vi "Tosca-Trace-Logging Thread.vi"(7 "IPC":T1) -> ()   [LabVIEW 2020]
uses:
  IPC VIs/Tosca-IPC.ctl
  Classes/Parameters/Parameters.lvclass
  Digital Input VIs/Tosca-DI Queue Data.ctl
  Digital Input VIs/Tosca-Input Event.ctl
  Digital Input VIs/Tosca-Input Criterion.ctl
  epl-vi-lib/Utility VIs/Type Defs/Logic State.ctl
  Typedefs/Tosca-Accumulator.ctl
  Typedefs/Tosca-State AODO.ctl
  Typedefs/Tosca-AO Runtime.ctl
  Typedefs/Tosca-DO Runtime.ctl
  epl-vi-lib/Signal Synthesis VIs/4th Generation/Classes/SignalManager/SignalManager.lvclass
  Typedefs/Tosca-Synapse Start Data.ctl
  IPC VIs/Tosca-Message.ctl
  IPC VIs/Tosca-Message Action.ctl
  Typedefs/Tosca-Thread Type.ctl
  Imaging VIs/Tosca-2P-Notifier Data.ctl
  Typedefs/Tosca-MATLAB Queue Data.ctl
  Visual Stim VIs/Tosca-Grating.ctl
  Visual Stim VIs/Tosca-Grating Type.ctl
  Typedefs/Tosca-File IO Notification.ctl
  Tosca-Trace Data.ctl
  Tosca-Trace-Event.ctl
  <vilib>/Utility/error.llb/Error Cluster From Error Code.vi
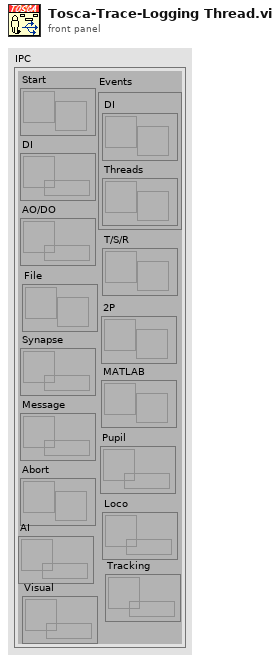
[diagram p1: front panel]
types:
  T1 = typedef "Tosca-IPC.ctl" = cluster{"Start":refnum<notifier>, "DI":refnum<queue>, "AO/DO":refnum<queue>, "Synapse":refnum<queue>, "Message":refnum<queue>, "Abort":refnum<notifier>, "Events":cluster{"DI":refnum<user-event>, "Threads ":refnum<user-event>}, "T/S/R":refnum<notifier>, "2P":refnum<notifier>, "MATLAB":refnum<notifier>, "Pupil":refnum<queue>, "Loco":refnum<queue>, "AI":refnum<queue>, "Tracking":refnum<queue>, "Visual":refnum<queue>, "File":refnum<notifier>}
  T2 = typedef "Tosca-Trace Data.ctl" = cluster{"Time":dbl, "Event":T3, "Source":string, "Message":string, "Data":dbl}
  T3 = typedef "Tosca-Trace-Event.ctl" = enum16{"Unspecified", "Trial start", "Enqueue", "Result", "End parser", "Frame", "Queue available", "Timeout sent", "WritePos", "TTL"}
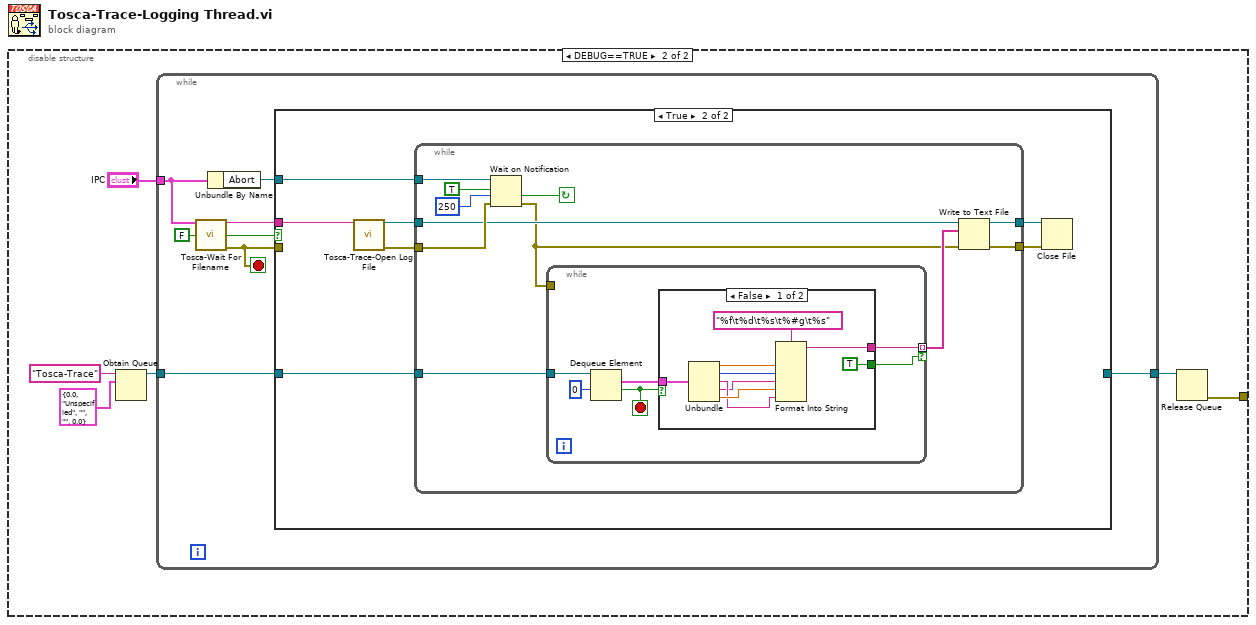
[diagram p0: block diagram]
diagram:
  n1 = disable-structure shown="DEBUG==TRUE" {
    disable-tunnel: [_ w1] -> _
    frame condition #0 {
    }
    frame condition #1 (active) {
      n2 = Obtain Queue(name (unnamed)="Tosca-Trace", element data type=T2 {"Time"=0.0, "Event"=enum."Unspecified", "Source"="", "Message"="", "Data"=0.0} ("Trace Data")) -> (queue out=w3:refnum<queue>)  [unwired: 3 in, 2 out]
      n3 = while {
        tunnel: w3 -> [w14]
        tunnel: [w13] -> w6
        tunnel: "IPC" -> [w10]
        stop <- w8 stop-if-true
        n4 = call "Tosca-Wait For Filename.vi"("IPC"=w10, "Times out?"=FALSE ("Time out?")) -> ("Filestem"=w12:string, "Received"=w11:bool, "error out"=w8:errorcluster)  [unwired: 11 in]
        n5 = Unbundle By Name(w10) -> ("Abort"=w9:refnum<notifier>)
        n6 = case shown="True" w11 {
          tunnel: w12 -> [_ w16]
          tunnel: w14 -> [w15 w20]
          tunnel: w9 -> [_ w21]
          tunnel: [w15 _] -> w13
          tunnel: w8 -> [_ _]
          frame False {
          }
          frame True {
            n7 = call "Tosca-Trace-Open Log File.vi"("Filestem"=w16) -> ("refnum out"=w22:refnum<file>, "error out"=w19:errorcluster)  [unwired: 13 in]
            n8 = while {
              tunnel: w22 -> [w29]
              tunnel: w21 -> [w33]
              tunnel: w20 -> [w31]
              tunnel: w19 -> [w30]
              tunnel: [w25] -> w17
              tunnel: [w24] -> w18
              stop <- w26 continue-if-true
              n9 = Wait on Notification(notifier=w33, ignore previous (F)=TRUE, timeout in ms (-1)=250, error in (no error)=w30) -> (timed out?=w26:bool, error out=w27:errorcluster)  [unwired: 2 out]
              n10 = while {
                tunnel: w31 -> [w39]
                tunnel: [w36] -> w28 mode=indexing if=w34
                tunnel: w27 -> [_]
                stop <- w35 stop-if-true
                n11 = Dequeue Element(queue=w39, timeout in ms (-1)=0) -> (element=w37:T2, timed out?=w35:bool)  [unwired: 1 in, 2 out]
                n12 = case shown="False" w35 {
                  tunnel: w37 -> [w48 _]
                  tunnel: [w44 _] -> w36
                  tunnel: [TRUE _] -> w34
                  frame False {
                    n13 = Unbundle(w48) -> ("Time"=w46:dbl, "Event"=w45:T3, "Source"=w41:string, "Message"=w40:string, "Data"=w42:dbl)
                    n14 = Format Into String(format string="%f\t%d\t%s\t%#g\t%s", w46, w45, w40, w42, w41) -> (resulting string=w44:string)  [unwired: 2 in, 1 out]
                  }
                  frame True {
                  }
                }
              }
              n15 = Write to Text File(file (use dialog)=w29, text=w28, error in=w27) -> (refnum out=w25:refnum<file>, error out=w24:errorcluster)  [unwired: 1 in, 1 out]
            }
            n16 = Close File(refnum=w17, error in=w18) -> ()  [unwired: 2 out]
          }
        }
      }
      n17 = Release Queue(queue=w6) -> (error out=w1:errorcluster)  [unwired: 2 in, 2 out]
    }
  }
